vi "Cache_Path Global_Read.vi"(5 "Show UI?(F)":bool, 7 "Interrupt":refnum<notifier>, 8 "error in (no error)":errorcluster, 11 "Class Name":string) -> (0 "error out":errorcluster, 1 "Success?":bool, 3 "Class Path":path)   [LabVIEW 2020, in "ClassLoader.lvlib"]
uses:
  ClassLoader.lvlib
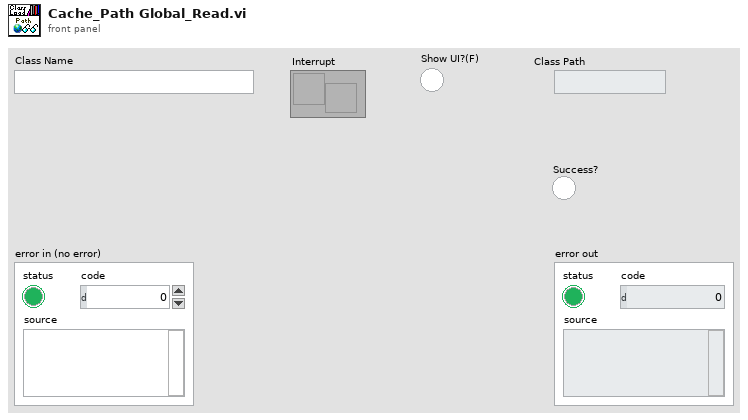
[diagram p1: front panel]
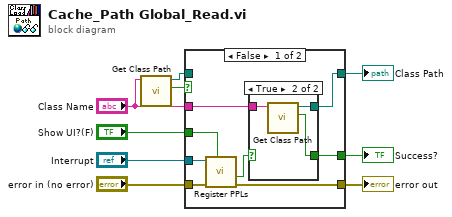
[diagram p0: block diagram]
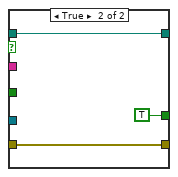
[diagram p3: hidden frame]
diagram:
  n1 = call "Get Class Path.vi"("Class Name"="Class Name") -> ("Success?"=w1:bool, "Path"=w2:path)  [unwired: 9 in]
  n2 = case shown="False" w1 {
    tunnel: "error in (no error)" -> [w17 w22]
    tunnel: "Class Name" -> [w15 _]
    tunnel: [w13 w24] -> w8
    tunnel: w2 -> [_ w24]
    tunnel: [w14 TRUE] -> w7
    tunnel: [w12 w22] -> w6
    tunnel: "Show UI?(F)" -> [w11 _]
    tunnel: "Interrupt" -> [w10 _]
    frame False {
      n3 = call "Register PPLs.vi"("Show UI?(F)"=w11, "error in"=w17, "Interrupt"=w10) -> ("error out"=w12:errorcluster, "Success?"=w16:bool)  [unwired: 7 in]
      n4 = case shown="True" w16 {
        selector: w16 -> [w18 _]
        tunnel: w15 -> [_ w21]
        tunnel: [w18 w20] -> w14
        tunnel: [_ w19] -> w13
        frame False {
        }
        frame True {
          n5 = call "Get Class Path.vi"("Class Name"=w21) -> ("Success?"=w20:bool, "Path"=w19:path)  [unwired: 9 in]
        }
      }
    }
    frame True {
    }
  }
  "error out" <- w6
  "Class Path" <- w8
  "Success?" <- w7
